vi "AutoJump.vi"(9 "Current Index":i32, 11 "Array":dbl[](array[numeric]) format="%0.3f") -> (1 "New Index":i32)   [LabVIEW 2013]
uses:
  Robot Global Data.vi
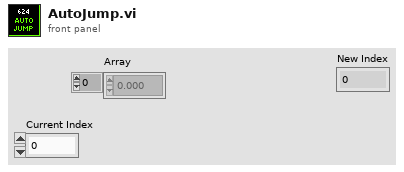
[diagram p1: front panel]
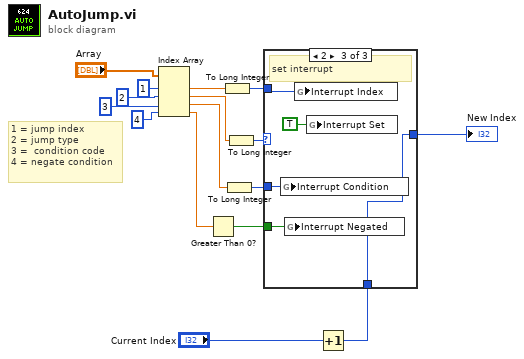
[diagram p0: block diagram]
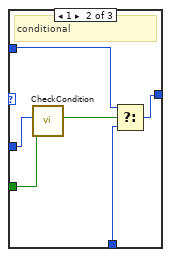
[diagram p3: hidden frame]
diagram:
  # "1 = jump index\n2 = jump type\n3 =  condition code\n4 = negate condition"
  n1 = Index Array(array="Array", index #1=1 ("index"), index #2=2 ("index"), index #3=3 ("index"), index #4=4 ("index")) -> (element #1=w13:dbl, element #2=w5:dbl, element #3=w4:dbl, element #4=w3:dbl)
  n2 = Greater Than 0?(x=w3) -> (x > 0?=w1:bool)
  n3 = To Long Integer(number=w13) -> (32bit integer=w12:i32)
  n4 = To Long Integer(number=w4) -> (32bit integer=w10:i32)
  n5 = To Long Integer(number=w5) -> (32bit integer=w11:i32)
  n6 = Increment(x="Current Index") -> (x+1=w8:i32)
  n7 = case shown="2" w11 {
    tunnel: w12 -> [w17 w20 w26]
    tunnel: w10 -> [_ w23 w25]
    tunnel: w8 -> [_ w22 w28]
    tunnel: [w17 w21 w28] -> w14
    tunnel: w1 -> [_ w18 w24]
    frame 0, Default {
      # "unconditional"
    }
    frame 1 {
      # "conditional"
      n8 = call "CheckCondition.vi"("Negate"=w18, "Condition"=w23) -> ("Condition True?"=w19:bool)  [unwired: 9 in]
      n9 = Select(t=w20, s=w19, f=w22) -> (s? t:f=w21:i32)
    }
    frame 2 {
      # "set interrupt"
      n10 = global write "Robot Global Data.vi" "Interrupt Condition"(w25) -> ()
      n11 = global write "Robot Global Data.vi" "Interrupt Negated"(w24) -> ()
      n12 = global write "Robot Global Data.vi" "Interrupt Index"(w26) -> ()
      n13 = global write "Robot Global Data.vi" "Interrupt Set"(TRUE ("Interrupt Set")) -> ()
    }
  }
  "New Index" <- w14
